vi "PQexecParams.vi"(0 "nParams":u64, 1 "command":string, 2 "conn":u64, 5 "paramTypes":u64[](array[numeric]), 7 "paramLengths":u64[](array[numeric]), 9 "paramFormats":u64[](array[numeric]), 11 "paramValues":string[](array[string]), 12 "resultFormat":u64, 13 "error in (no error)":errorcluster) -> (4 "conn_out":u64, 8 "res":u64, 15 "error out":errorcluster)   [LabVIEW 2019, in "libpqlv64.lvlib"]
doc: "Submits a command to the server and waits for the result, with the ability to pass parameters separately from the SQL command text.\n\nhttp://www.postgresql.org/docs/8.1/interactive/libpq-exec.html"
uses:
  libpqlv64.lvlib
  libpq.dll
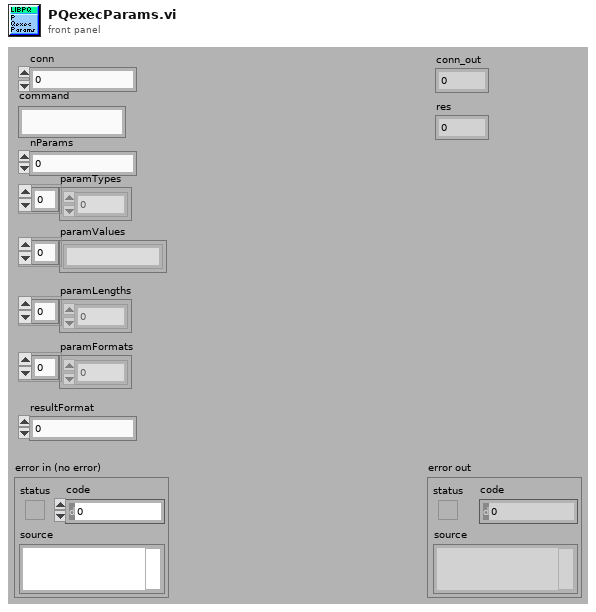
[diagram p1: front panel]
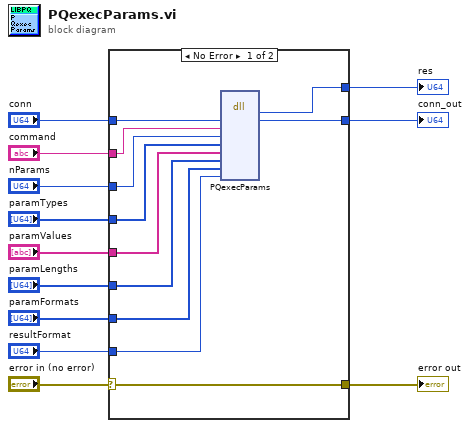
[diagram p0: block diagram]
diagram:
  n1 = case shown="No Error" "error in (no error)" {
    selector: "error in (no error)" -> [w23 w25]
    tunnel: [w23 w25] -> w11
    tunnel: [w22 _] -> w10
    tunnel: "command" -> [w21 _]
    tunnel: "nParams" -> [w20 _]
    tunnel: "paramTypes" -> [w19 _]
    tunnel: "paramValues" -> [w16 _]
    tunnel: "paramLengths" -> [w18 _]
    tunnel: "resultFormat" -> [w17 _]
    tunnel: "conn" -> [w15 w24]
    tunnel: [w14 w24] -> w4
    tunnel: "paramFormats" -> [w13 _]
    frame No Error {
      n2 = dll-call lib="libpq.*" fn="PQexecParams"("conn"=w15, "command"=w21, "nParams"=w20, "paramTypes"=w19, "paramValues"=w16, "paramLengths"=w18, "paramFormats"=w13, "resultFormat"=w17) -> ("res"=w22:u64, "conn"=w14:u64)  [unwired: 10 in, 2 out]
    }
    frame Error {
    }
  }
  "res" <- w10
  "error out" <- w11
  "conn_out" <- w4
